vi "begin drive train subVI.vi"   [LabVIEW 2017]
uses:
  <vilib>/Rock Robotics/WPI/SafetyOutput/WPI_SafetyOutputConfigMenu.ctl
  <vilib>/Rock Robotics/WPI/RobotDrive/WPI_RobotDriveOpen2MotorWithExistingMotors.vi
types:
  T1 = typedef "WPI_SafetyOutputConfigMenu.ctl" = enum16{"Enable", "Disable"}
  T2 = typedef "WPI_MotorControlDeviceRef.ctl" = cluster{"DeviceStatus":errorcluster, "Type":T3, "PWM":cluster{"PWM Channel":T4, "DeadBand":T5}, "CAN":cluster{"Device Number":u8, "SetOutput VI Ref":variant, "GetOutput VI Ref":variant, "Enable VI Ref":variant, "Disable VI Ref":variant, "Data":variant}, "Invert":bool, "DIO PWM":cluster{"PWM \"Enable\" Channel":T4, "DIOChannel":T6, "PWM Rate":dbl}}
  T3 = typedef "WPI_MotorControlType.ctl" = enum16{"PWM", "CAN", "DIO PWM"}
  T4 = typedef "FPGA_DIOPWMChannel.ctl" = enum8{"PWM 0", "PWM 1", "PWM 2", "PWM 3", "PWM 4", "PWM 5", "PWM 6", "PWM 7", "PWM 8", "PWM 9", "PWM MXP 0", "PWM MXP 1", "PWM MXP 2", "PWM MXP 3", "PWM MXP 4", "PWM MXP 5", "PWM MXP 6", "PWM MXP 7", "PWM MXP 8", "PWM MXP 9", "Invalid"}
  T5 = typedef "WPI_PWMDeadband.ctl" = cluster{"Name":string, "maxPositivePwm":i32, "minPositivePwm":i32, "centerPwm":i32, "maxNegativePwm":i32, "minNegativePwm":i32, "angularRange":u16}
  T6 = typedef "FPGA_DIOChannel.ctl" = enum8{"DIO 0", "DIO 1", "DIO 2", "DIO 3", "DIO 4", "DIO 5", "DIO 6", "DIO 7", "DIO 8", "DIO 9", "DIO MXP 0", "DIO MXP 1", "DIO MXP 2", "DIO MXP 3", "DIO MXP 4", "DIO MXP 5", "DIO MXP 6", "DIO MXP 7", "DIO MXP 8", "DIO MXP 9", "DIO MXP 10", "DIO MXP 11", "DIO MXP 12", "DIO MXP 13", "DIO MXP 14", "DIO MXP 15", "SPI Port CS1", "SPI Port CS2", "SPI Port CS3", "SPI Port MISO", "SPI Port MOSI", "Invalid"}
  T7 = typedef "WPI_RobotDriveDevRef.ctl" = cluster{"DevStatus":errorcluster, "Motors[]":T2[], "Square Inputs":bool, "Max Output":dbl}
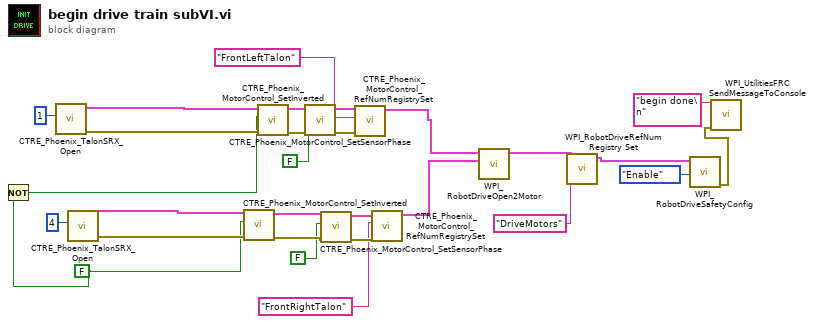
[diagram p0: block diagram]
diagram:
  w21 = FALSE ("Invert?")
  n1 = Not(x=w21) -> (.not. x?=w22:bool)
  n2 = call <vilib>:"CTRE_Phoenix_TalonSRX_Open.vi"("Device Number"=u8 1) -> ("error out"=w24:errorcluster, "CAN Talon SRX Ref"=w23:T2)  [unwired: 9 in]
  n3 = call <vilib>:"CTRE_Phoenix_TalonSRX_Open.vi"("Device Number"=u8 4) -> ("error out"=w26:errorcluster, "CAN Talon SRX Ref"=w25:T2)  [unwired: 9 in]
  n4 = call <vilib>:"CTRE_Phoenix_MotorControl_SetInverted.vi"("error in (no error)"=w26, "Invert?"=w21, "PhoenixMotorControlDevRef"=w25) -> ("error out"=w20:errorcluster, "PhoenixMotorControlDevRef"=w19:T2)  [unwired: 7 in]
  n5 = call <vilib>:"CTRE_Phoenix_MotorControl_SetInverted.vi"("error in (no error)"=w24, "Invert?"=w22, "PhoenixMotorControlDevRef"=w23) -> ("error out"=w18:errorcluster, "PhoenixMotorControlDevRef"=w17:T2)  [unwired: 7 in]
  n6 = call <vilib>:"CTRE_Phoenix_MotorControl_SetSensorPhase.vi"("error in (no error)"=w18, "PhaseSensor"=FALSE, "PhoenixMotorControlDevRef"=w17) -> ("error out"=w11:errorcluster, "PhoenixMotorControlDevRef"=w12:T2)  [unwired: 7 in]
  n7 = call <vilib>:"CTRE_Phoenix_MotorControl_SetSensorPhase.vi"("error in (no error)"=w20, "PhaseSensor"=FALSE, "PhoenixMotorControlDevRef"=w19) -> ("error out"=w10:errorcluster, "PhoenixMotorControlDevRef"=w9:T2)  [unwired: 7 in]
  n8 = call <vilib>:"CTRE_Phoenix_MotorControl_RefNumRegistrySet.vi"("error in (no error)"=w11, "refnum name"="FrontLeftTalon", "PhoenixMotorControlDevRef"=w12) -> ("PhoenixMotorControlDevRef"=w13:T2)  [unwired: 7 in, 1 out]
  n9 = call <vilib>:"CTRE_Phoenix_MotorControl_RefNumRegistrySet.vi"("error in (no error)"=w10, "refnum name"="FrontRightTalon", "PhoenixMotorControlDevRef"=w9) -> ("PhoenixMotorControlDevRef"=w14:T2)  [unwired: 7 in, 1 out]
  n10 = call-poly <vilib>:"WPI_RobotDriveOpen2Motor.vi"("Right Motor Dev Ref"=w14, "Left Motor Dev Ref"=w13) -> ("RobotDriveDevRef"=w3:T7)  [unwired: 8 in, 1 out]
  n11 = call <vilib>:"WPI_RobotDriveRefNum Registry Set.vi"("refnum name"="DriveMotors", "RobotDriveDevRef"=w3) -> ("RobotDriveDevRef"=w6:T7)  [unwired: 8 in, 1 out]
  n12 = call <vilib>:"WPI_RobotDriveSafetyConfig.vi"("mode"=WPI_SafetyOutputConfigMenu."Enable", "RobotDriveDevRef"=w6) -> ("error out"=w27:errorcluster)  [unwired: 8 in, 1 out]
  n13 = call <vilib>:"WPI_UtilitiesFRC SendMessageToConsole.vi"("Message"="begin done\n", "error in (no error)"=w27) -> ()  [unwired: 13 in, 1 out]
